vi "deadband.vi"(7 "minAbsX":dbl, 10 "x":dbl) -> (2 "x out":dbl)   [LabVIEW 2010]
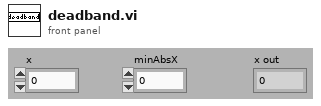
[diagram p1: front panel]
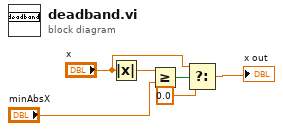
[diagram p0: block diagram]
diagram:
  n1 = Absolute Value(x="x") -> (abs(x)=w6:dbl)
  n2 = Greater Or Equal?(x=w6, y="minAbsX") -> (x >= y?=w4:bool)
  n3 = Select(t="x", s=w4, f=0.0) -> (s? t:f=→"x out":dbl)
